vi "Initiate Trigger.vi"(8 "error in (no error)":errorcluster, 9 "Enable Continuous Transient Trigger (T: Enable)":bool=TRUE, 10 "Trigger Type (0:Transient)":u16(ring) items=["Transient", "Acquire"], 11 "VISA resource name":refnum<visa-resource-name>) -> (0 "error out":errorcluster, 3 "VISA resource name out":refnum<visa-resource-name>)   [LabVIEW 2010, in "California Instruments iX Series.lvlib"]
doc: "Initiates a measurement based on the preset configuration. The measurement type must be configured before calling this function. This is accomplished by calling the <b>Configure Trigger VI</b>. After the Initiate VI is called, the instrument leaves the Idle state and waits for a trigger."
uses:
  <instrlib>/California Instruments iX Series/California Instruments iX Series.lvlib
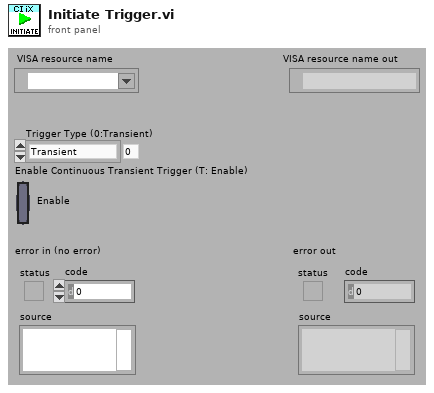
[diagram p1: front panel]
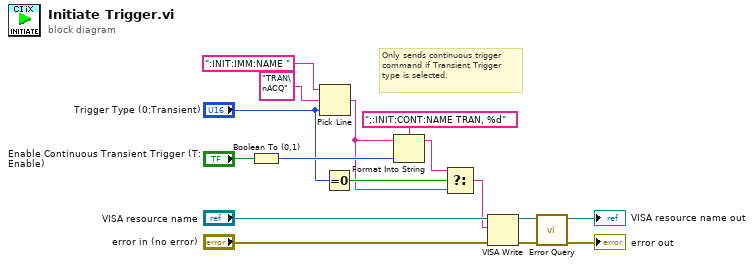
[diagram p0: block diagram]
diagram:
  # "Only sends continuous trigger command if Transient Trigger type is selected."
  n1 = Boolean To (0,1)(Boolean="Enable Continuous Transient Trigger (T: Enable)") -> (0, 1=w6:i16)
  n2 = Pick Line(string ("")=":INIT:IMM:NAME ", multi-line string="TRAN\nACQ", line index="Trigger Type (0:Transient)") -> (output string=w2:string)
  n3 = Equal To 0?(x="Trigger Type (0:Transient)") -> (x = 0?=w8:bool)
  n4 = Format Into String(format string=";:INIT:CONT:NAME TRAN, %d", initial string=w2, w6) -> (resulting string=w3:string)  [unwired: 1 in, 1 out]
  n5 = Select(t=w3, s=w8, f=w2) -> (s? t:f=w1:string)
  n6 = VISA Write(VISA resource name="VISA resource name", write buffer=w1, error in (no error)="error in (no error)") -> (VISA resource name out=w14:refnum<visa-resource-name>, error out=w13:errorcluster)  [unwired: 1 out]
  n7 = call <instrlib>:"Error Query.vi"("error in (no error)"=w13, "VISA resource name"=w14) -> ("error out"=→"error out":errorcluster, "VISA resource name out"=→"VISA resource name out":refnum<visa-resource-name>)  [unwired: 6 in, 2 out]
